vi "MEASUREMENT FUNCTION.vi"(0 "VISA resource name":refnum<visa-resource-name>="GPIB0::1::INSTR", 1 "CHANNEL":enum32{"CH 1", "CH 2", "CH 3", "CH 4"}(radio), 2 "MEASU":T2(ring), 3 "MEAS TYPEs":T1(ring)) -> (8 "MEAS VALUE":string)   [LabVIEW 2011]
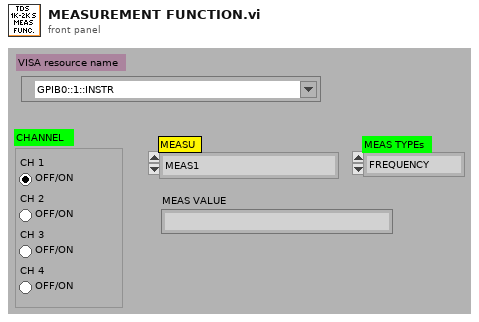
[diagram p1: front panel]
types:
  T1 = enum16{"FREQUENCY", "MEAN", "PERIOD", "PK2PK", "MIN", "MAX", "RISE", "FALL", "CRMS", "PWIDTH", "NWIDTH", "NONE"}
  T2 = enum16{"MEAS1", "MEAS2", "MEAS3", "MEAS4", "MEAS5"}
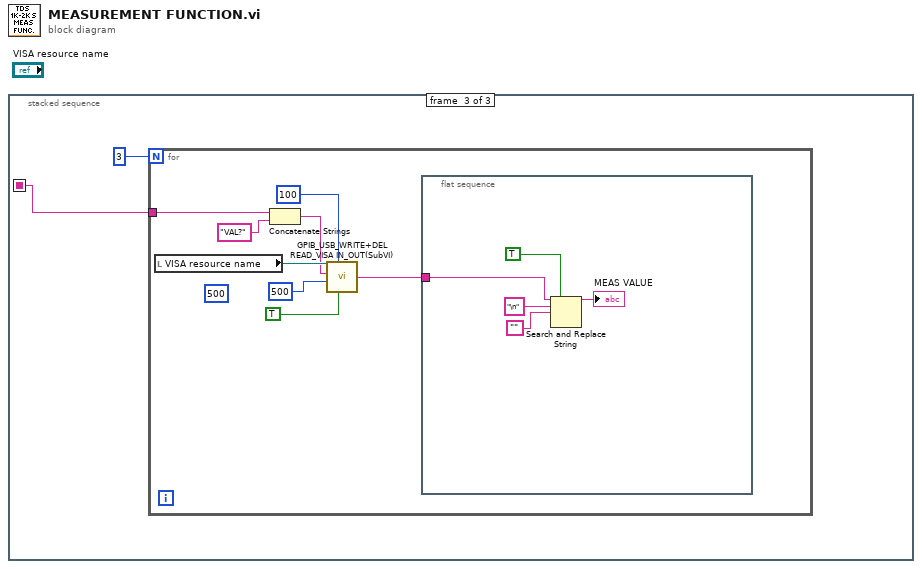
[diagram p0: block diagram]
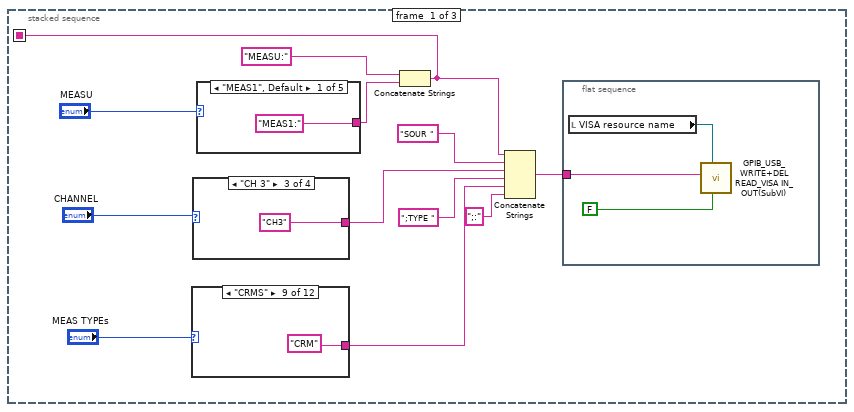
[diagram p2: hidden frame]
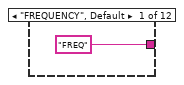
[diagram p3: hidden frame]
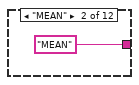
[diagram p4: hidden frame]
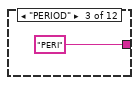
[diagram p5: hidden frame]
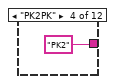
[diagram p6: hidden frame]
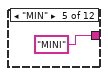
[diagram p7: hidden frame]
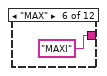
[diagram p8: hidden frame]
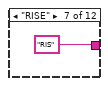
[diagram p9: hidden frame]
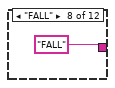
[diagram p10: hidden frame]
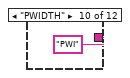
[diagram p11: hidden frame]
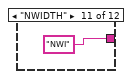
[diagram p12: hidden frame]
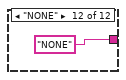
[diagram p13: hidden frame]
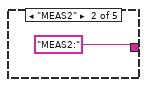
[diagram p14: hidden frame]
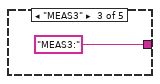
[diagram p15: hidden frame]
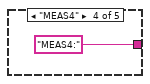
[diagram p16: hidden frame]
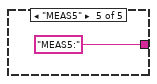
[diagram p17: hidden frame]
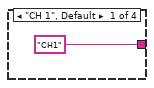
[diagram p18: hidden frame]
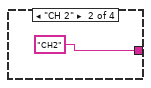
[diagram p19: hidden frame]
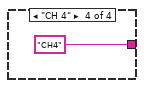
[diagram p20: hidden frame]
diagram:
  n1 = stacked-sequence {
    seq-local: [w1 _ _] -> [_ _ w39]
    frame #0 {
      n2 = case shown="\"CRMS\"" "MEAS TYPEs" {
        tunnel: ["FREQ" "MEAN" "PERI" "PK2" "MINI" "MAXI" "RIS" "FALL" "CRM" "PWI" "NWI" "NONE"] -> w6
        frame "FREQUENCY", Default {
        }
        frame "MEAN" {
        }
        frame "PERIOD" {
        }
        frame "PK2PK" {
        }
        frame "MIN" {
        }
        frame "MAX" {
        }
        frame "RISE" {
        }
        frame "FALL" {
        }
        frame "CRMS" {
        }
        frame "PWIDTH" {
        }
        frame "NWIDTH" {
        }
        frame "NONE" {
        }
      }
      n3 = case shown="\"CH 3\"" "CHANNEL" {
        tunnel: ["CH1" "CH2" "CH3" "CH4"] -> w9
        frame "CH 1", Default {
        }
        frame "CH 2" {
        }
        frame "CH 3" {
        }
        frame "CH 4" {
        }
      }
      n4 = case shown="\"MEAS1\", Default" "MEASU" {
        tunnel: ["MEAS1:" "MEAS2:" "MEAS3:" "MEAS4:" "MEAS5:"] -> w3
        frame "MEAS1", Default {
        }
        frame "MEAS2" {
        }
        frame "MEAS3" {
        }
        frame "MEAS4" {
        }
        frame "MEAS5" {
        }
      }
      n5 = Concatenate Strings("MEASU:", w3) -> (w1:string)
      n6 = Concatenate Strings(w1, "SOUR ", w9, ";TYPE ", w6, ";:") -> (w4:string)
      n7 = flat-sequence {
        tunnel: w4 -> [w15]
        frame #0 {
          n8 = local read "VISA resource name"() -> (w14:refnum<visa-resource-name>)
          n9 = call "GPIB_USB_WRITE+DEL READ_VISA IN_OUT(SubVI).vi"("VISA resource IN"=w14, "GPIB/USB WRITE"=w15, 4:FALSE ("READ GPIB")) -> ()  [unwired: 3 in, 3 out]
        }
      }
    }
    frame #1 {
      # "500"
      n10 = flat-sequence {
        frame #0 {
          n11 = Wait (ms)(milliseconds to wait=u32 400) -> ()  [unwired: 1 out]
        }
      }
    }
    frame #2 {
      n12 = for {
        N: 3 -> [_]
        tunnel: w39 -> [w47]
        (unwired) u32 500 ("DELAY BEFORE READ")
        n13 = local read "VISA resource name"() -> (w46:refnum<visa-resource-name>)
        n14 = Concatenate Strings(w47, "VAL?") -> (w42:string)
        n15 = call "GPIB_USB_WRITE+DEL READ_VISA IN_OUT(SubVI).vi"("VISA resource IN"=w46, "BYTE COUNT"=u32 100 ("Byte count"), "GPIB/USB WRITE"=w42, "DELAY BEFORE READ"=u32 500, 4:TRUE ("READ GPIB")) -> ("GPIB/USB READ"=w41:string)  [unwired: 1 in, 2 out]
        n16 = flat-sequence {
          tunnel: w41 -> [w48]
          frame #0 {
            n17 = Search and Replace String(replace all?=TRUE ("replace all? (F)"), input string=w48, search string="\n", replace string="") -> (result string=→"MEAS VALUE":string)  [unwired: 1 in, 6 out]
          }
        }
      }
    }
  }
